vi "PTv3.0.vi"(8 "error in":errorcluster) -> ()   [LabVIEW 2017]
doc: "This VI runs in parallel to other tasks. It can contain as many user-defined periodic loops as you need. These can carry out PID or other sorts of timed response."
uses:
  <vilib>/Rock Robotics/WPI/DriverStation/WPI_DriverStationRobotMode2.ctl
  <vilib>/Analysis/baseanly.llb/Mean (DBL).vi
  <vilib>/Rock Robotics/WPI/Utilities/WPI_GetSetVariantRefNum.vi
  <vilib>/Rock Robotics/Network Tables/NT Read Boolean.vi
  <vilib>/Rock Robotics/Network Tables/NT Read Number.vi
  Robot Global Data.vi
  <vilib>/Rock Robotics/Network Tables/NT Write Number.vi
  <vilib>/Rock Robotics/Network Tables/NT Write Numeric Array.vi
  <vilib>/Analysis/NI_AALBase.lvlib
panel:
  out "Arrayval":dbl
  out "Accelerations":T1
  out "Avg Y":dbl
  out "Current Joy Y Value":dbl
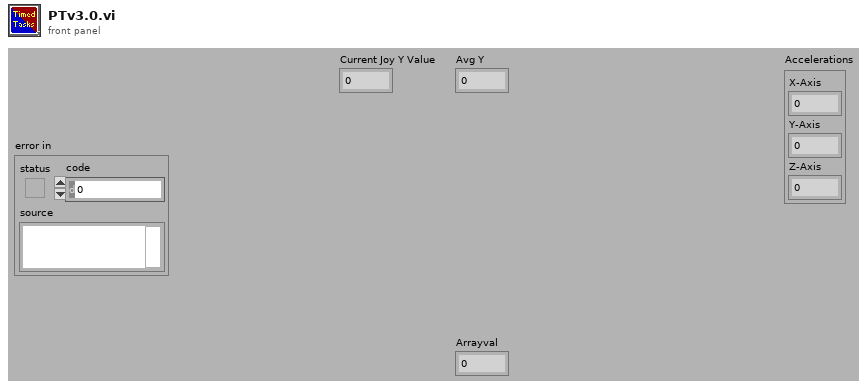
[diagram p1: front panel]
types:
  T1 = cluster{"X-Axis":dbl, "Y-Axis":dbl, "Z-Axis":dbl}
  T2 = typedef "WPI_JoystickDevRef.ctl" = cluster{"Device":T3}
  T3 = typedef "WPI_JoystickDeviceEnum.ctl" = enum16{"USB 0", "USB 1", "USB 2", "USB 3", "USB 4", "USB 5"}
  T4 = typedef "WPI_GyroDevRef.ctl" = cluster{"DevStatus":errorcluster, "Analog Channel":T5, "Gain (VoltsPerDegree/Second)":dbl, "Gyro Type":enum16{"Analog", "XRS450"}, "Handle":i32, "SPI Bus":T6, "Device Found":bool, "Sample Rate":dbl, "Calibrate On Open":bool, "Offset":dbl}
  T5 = typedef "FPGA_AIChannel.ctl" = enum8{"AI 0", "AI 1", "AI 2", "AI 3", "AI MXP 0", "AI MXP 1", "AI MXP 2", "AI MXP 3", "Invalid"}
  T6 = typedef "spi_bus.ctl" = enum16{"SPI On-Board, CS0", "SPI On-Board, CS1", "SPI On-Board, CS2", "SPI On-Board, CS3", "SPI MXP", "Invalid"}
  T7 = typedef "WPI_AccelerometerDevRef.ctl" = cluster{"DevStatus":errorcluster, "Scaling":T8, "Analog Channels":T9, "I2C Bus":T10, "SPI Bus":T6, "Accel Range":T11, "ADXL Axes":T12, "Handle":i32, "Device Address":u8, "Accel Type":enum16{"Analog", "ADXL345 I2C", "ADXL345 SPI", "Internal", "ADXL362 SPI"}}
  T8 = typedef "WPI_AccelerometerScaling.ctl" = cluster{"Gain (VoltsPerG)":dbl, "Center Voltage":dbl}
  T9 = typedef "WPI_AccelerometerAnalogChannels.ctl" = cluster{"X-Axis":T5, "Y-Axis":T5, "Z-Axis":T5}
  T10 = typedef "i2c_bus.ctl" = enum16{"I2C On-Board", "I2C MXP", "Invalid"}
  T11 = typedef "ADXL345 Range.ctl" = u8
  T12 = typedef "WPI_AccelerometerADXL345 Axes.ctl" = cluster{"X-Axis":bool, "Y-Axis":bool, "Z-Axis":bool}
  T13 = typedef "WPI_DriverStationRobotMode2.ctl" = enum16{"Autonomous Disabled", "Autonomous Enabled", "Teleop Disabled", "Teleop Enabled", "Disconnected", "Finish", "Test Disabled", "Test Enabled", "Emergency Stopped"}
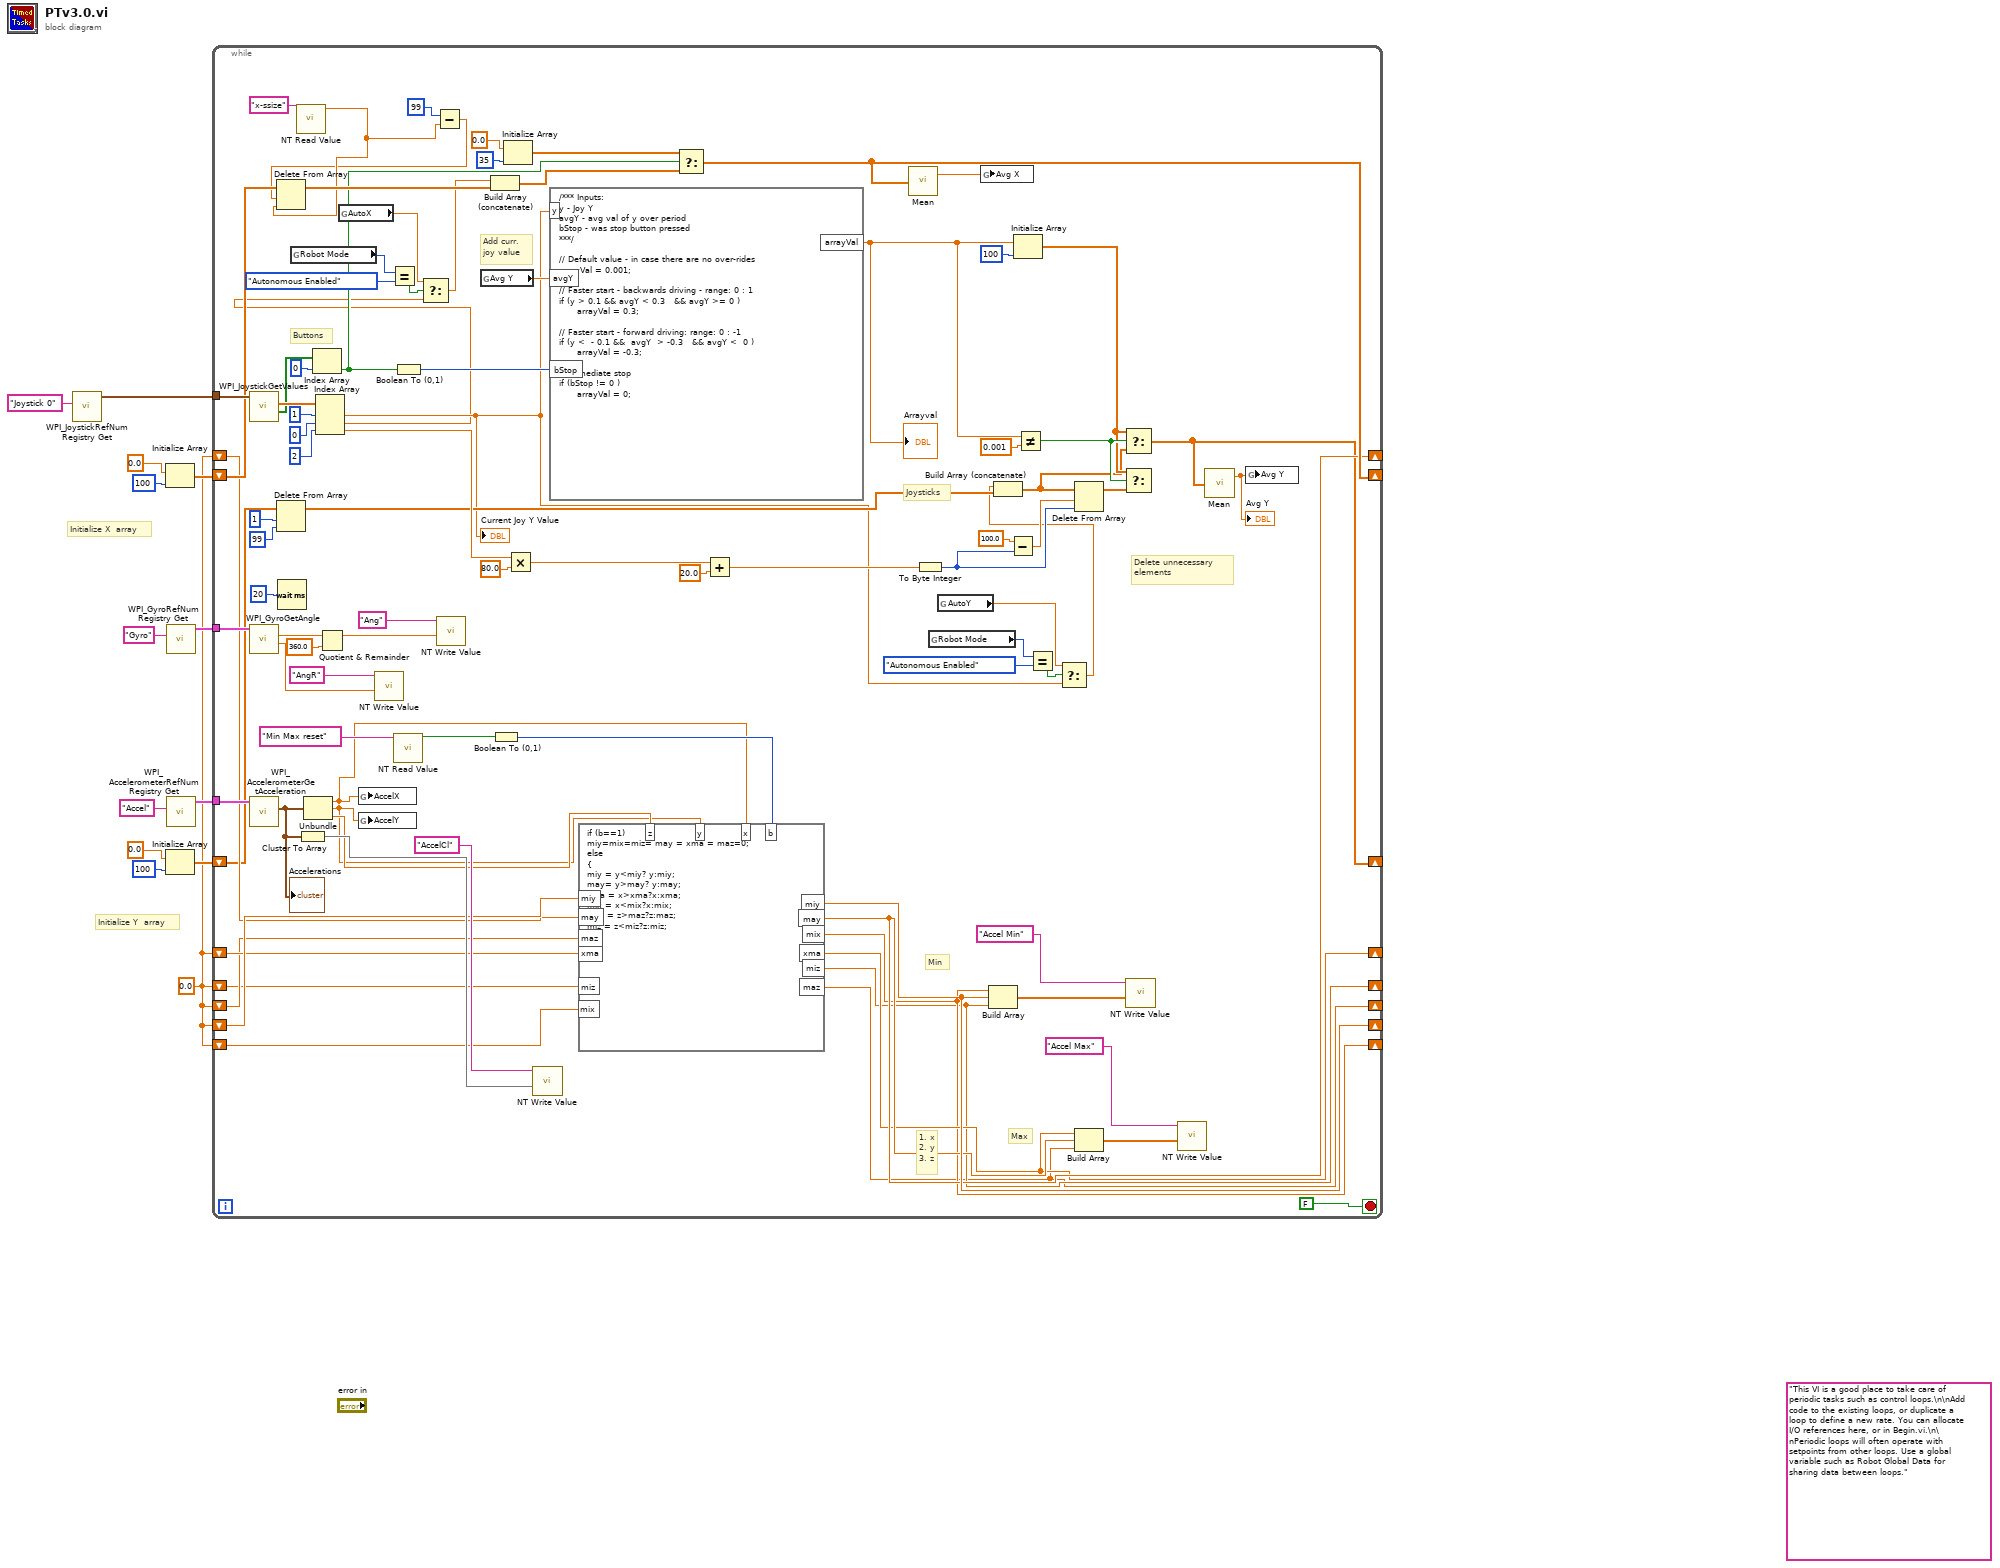
[diagram p0: block diagram]
diagram:
  w1 = 0.0 ("Y-Axis")
  (unwired) "This VI is a good place to take care of periodic tasks such as control loops.\n\nAdd code to the existing loops, or duplicate a loop to define a new rate. You can allocate I/O references here, or in Begin.vi.\n\nPeriodic loops will often operate with setpoints from other loops. Use a global variable such as Robot Global Data for sharing data between loops."
  # "Initialize X  array"
  # "Initialize Y  array"
  n1 = call <vilib>:"WPI_JoystickRefNum Registry Get.vi"("refnum name"="Joystick 0") -> ("JoystickDevRef"=w12:T2)  [unwired: 1 in, 9 out]
  n2 = Initialize Array(0.0 ("element"), 100 ("dimension size")) -> (w8:dbl[])
  n3 = Initialize Array(0.0 ("element"), 100 ("dimension size")) -> (w9:dbl[])
  n4 = call <vilib>:"WPI_GyroRefNum Registry Get.vi"("refnum name"="Gyro") -> ("GyroDevRef"=w2:T4)  [unwired: 9 in, 1 out]
  n5 = call <vilib>:"WPI_AccelerometerRefNum Registry Get.vi"("refnum name"="Accel") -> ("AccelerometerDevRef"=w4:T7)  [unwired: 9 in, 1 out]
  n6 = while {
    tunnel: w12 -> [w101]
    shift-right: [w18] -> _
    shift-left: w9 -> [w39]
    shift-right: [w95] -> _
    shift-left: w8 -> [w90]
    tunnel: w4 -> [w82]
    tunnel: w2 -> [w81]
    shift-right: [w59] -> _
    shift-left: w1 -> [w65]
    shift-right: [w60] -> _
    shift-left: w1 -> [w66]
    shift-right: [w56] -> _
    shift-left: w1 -> [w63]
    shift-right: [w58] -> _
    shift-left: w1 -> [w64]
    shift-right: [w61] -> _
    shift-left: w1 -> [w67]
    shift-right: [w57] -> _
    shift-left: w1 -> [w62]
    stop <- FALSE stop-if-true
    # "1. x\n2. y\n3. z"
    # "Max"
    # "Min"
    # "Add curr. \njoy value"
    # "Delete unnecessary \nelements"
    # "Joysticks"
    # "Buttons"
    n7 = call <vilib>:"WPI_JoystickGetValues.vi"("JoystickDevRef"=w101) -> ("Buttons"=w98:bool[], "Axes"=w100:dbl[])  [unwired: 6 in, 3 out]
    n8 = call <vilib>:"WPI_GyroGetAngle.vi"("GyroDevRef"=w81) -> ("Angular Rate"=w79:dbl, "Angle"=w74:dbl)  [unwired: 6 in, 3 out]
    n9 = call <vilib>:"WPI_AccelerometerGetAcceleration.vi"("AccelerometerDevRef"=w82) -> ("Accelerations"=w72:T1)  [unwired: 8 in, 2 out]
    "Accelerations" <- w72
    n10 = Delete From Array(array=w39, length=1, index=99) -> (array with subset deleted=w36:dbl[])  [unwired: 1 out]
    n11 = Wait (ms)(milliseconds to wait=u32 20) -> ()  [unwired: 1 out]
    n12 = global read "Robot Global Data.vi" "Robot Mode"() -> (w22:T13)
    n13 = call-poly <vilib>:"NT Read Value.vi"("Name"="x-ssize") -> ("Numeric"=w16:dbl)  [unwired: 9 in, 1 out]
    n14 = Cluster To Array(cluster=w72) -> (array=w80:dbl[])
    n15 = Unbundle(w72) -> ("X-Axis"=w32:dbl, "Y-Axis"=w31:dbl, "Z-Axis"=w68:dbl)
    n16 = Index Array(array=w98, index=0) -> (element=w85:bool)
    n17 = Index Array(array=w100, index #1=1 ("index"), index #2=0 ("index"), index #3=2 ("index")) -> (element #1=w27:dbl, element #2=w20:dbl, element #3=w41:dbl)
    "Current Joy Y Value" <- w27
    n18 = Quotient & Remainder(x=w74, y=360.0) -> (x-y*floor(x/y)=w73:dbl)  [unwired: 1 out]
    n19 = global read "Robot Global Data.vi" "AutoX"() -> (w19:dbl)
    n20 = global write "Robot Global Data.vi" "AccelX"(w32) -> ()
    n21 = global write "Robot Global Data.vi" "AccelY"(w31) -> ()
    n22 = call-poly <vilib>:"NT Write Value.vi"("Numeric"=w79, "Name"="AngR") -> ()  [unwired: 9 in, 1 out]
    n23 = Equal?(x=w22, y=WPI_DriverStationRobotMode2."Autonomous Enabled" ("Robot Mode")) -> (x = y?=w24:bool)
    n24 = Boolean To (0,1)(Boolean=w85) -> (0, 1=w86:i16)
    n25 = call-poly <vilib>:"NT Read Value.vi"("Name"="Min Max reset") -> ("Boolean"=w55:bool)  [unwired: 9 in, 1 out]
    n26 = Select(t=w19, s=w24, f=w20) -> (s? t:f=w21:dbl)
    n27 = Subtract(x=99, y=w16) -> (x-y=w15:dbl)
    n28 = Delete From Array(array=w90, length=w15, index=w16) -> (array with subset deleted=w91:dbl[])  [unwired: 1 out]
    n29 = call-poly <vilib>:"NT Write Value.vi"("Numeric"=w73, "Name"="Ang") -> ()  [unwired: 9 in, 1 out]
    n30 = global read "Robot Global Data.vi" "Avg Y"() -> (w87:dbl)
    n31 = Build Array (concatenate)(w21, w91) -> (w89:dbl[])
    n32 = Boolean To (0,1)(Boolean=w55) -> (0, 1=w54:i16)
    n33 = Initialize Array(0.0 ("element"), 35 ("dimension size")) -> (w94:dbl[])
    n34 = Multiply(x=w41, y=80.0) -> (x*y=w47:dbl)
    n35 = call-poly <vilib>:"NT Write Value.vi"("Numeric Array"=w80, "Name"="AccelCl") -> ()  [unwired: 9 in, 1 out]
    n36 = formula code="/*** Inputs:\ny - Joy Y\navgY - avg val of y over period\nbStop - was stop button pressed\n***/\n\n// Default value - in case there are no over-rides\narrayVal = 0.001;\n\n// Faster start - backwards driving - range: 0 : 1\nif (y > 0.1 && avgY < 0.3   && avgY >= 0 )\n      arrayVal = 0.3;\n\n// Faster start - forward driving: range: 0 : -1\nif (y <  - 0.1 &&  avgY  > -0.3   && avgY <  0 )\n      arrayVal = -0.3;\n\n// Immediate stop\nif (bStop != 0 )\n      arrayVal = 0;"("y"=w27, "avgY"=w87, "bStop"=w86) -> ("arrayVal"=w83:dbl)
    "Arrayval" <- w83
    n37 = formula code="if (b==1)\nmiy=mix=miz= may = xma = maz=0;\nelse \n{\nmiy = y<miy? y:miy;\nmay= y>may? y:may;\nxma = x>xma?x:xma;\nmix = x<mix?x:mix;\nmaz = z>maz?z:maz;\nmiz = z<miz?z:miz;\n}"("miy"=w67, "may"=w66, "x"=w32, "y"=w31, "z"=w68, "mix"=w64, "xma"=w65, "miz"=w62, "maz"=w63, "b"=w54) -> ("miy"=w61:dbl, "may"=w60:dbl, "mix"=w58:dbl, "xma"=w59:dbl, "miz"=w57:dbl, "maz"=w56:dbl)
    n38 = Select(t=w94, s=w85, f=w89) -> (s? t:f=w95:dbl[])
    n39 = Add(x=w47, y=20.0) -> (x+y=w45:dbl)
    n40 = call-poly <vilib>:"Mean.vi"("X"=w95) -> ("mean"=w71:dbl)  [unwired: 1 out]
    n41 = To Byte Integer(number=w45) -> (8bit integer=w43:i8)
    n42 = global read "Robot Global Data.vi" "Robot Mode"() -> (w30:T13)
    n43 = global read "Robot Global Data.vi" "AutoY"() -> (w25:dbl)
    n44 = global write "Robot Global Data.vi" "Avg X"(w71) -> ()
    n45 = Build Array(w58, w61, w57) -> (w52:dbl[])
    n46 = Subtract(x=100.0, y=w43) -> (x-y=w42:dbl)
    n47 = Initialize Array(w83, 100 ("dimension size")) -> (w34:dbl[])
    n48 = Not Equal?(x=w83, y=0.001) -> (x != y?=w35:bool)
    n49 = Equal?(x=w30, y=WPI_DriverStationRobotMode2."Autonomous Enabled" ("Robot Mode")) -> (x = y?=w28:bool)
    n50 = Select(t=w25, s=w28, f=w27) -> (s? t:f=w26:dbl)
    n51 = Build Array (concatenate)(w26, w36) -> (w33:dbl[])
    n52 = Delete From Array(array=w33, length=w42, index=w43) -> (array with subset deleted=w40:dbl[])  [unwired: 1 out]
    n53 = Build Array(w59, w60, w56) -> (w53:dbl[])
    n54 = Select(t=w34, s=w35, f=w33) -> (s? t:f=w18:dbl[])
    n55 = Select(t=w34, s=w35, f=w40) -> ()  [unwired: 1 out]
    n56 = call-poly <vilib>:"NT Write Value.vi"("Numeric Array"=w52, "Name"="Accel Min") -> ()  [unwired: 9 in, 1 out]
    n57 = call-poly <vilib>:"NT Write Value.vi"("Numeric Array"=w53, "Name"="Accel Max") -> ()  [unwired: 9 in, 1 out]
    n58 = call-poly <vilib>:"Mean.vi"("X"=w18) -> ("mean"=w70:dbl)  [unwired: 1 out]
    "Avg Y" <- w70
    n59 = global write "Robot Global Data.vi" "Avg Y"(w70) -> ()
  }
